vi "Test Open Close.vi"(8 "error in (no error)":errorcluster, 11 "Instrument.Oxford1820 in":refnum<class "Instrument.Oxford1820.lvclass">) -> (0 "error out":errorcluster, 3 "Instrument.Oxford1820 out":refnum<class "Instrument.Oxford1820.lvclass">)   [LabVIEW 2019, in "Instrument.Oxford1820.lvclass"]
uses:
  Instrument.Oxford1820.lvclass
  <instrlib>/Mercury iXX/Public/Libraries/Magnet/Controls/Device (Read).ctl
  <instrlib>/Mercury iXX/Public/Controls/Manufacturing Data.ctl
  <instrlib>/Mercury iXX/Public/Libraries/Magnet/Controls/Signals (Read).ctl
  Instrument.Oxford1820.lvclass/Instrument.Oxford1820.ctl
  <instrlib>/Mercury iXX/Public/Libraries/Magnet/Open/Open Magnet Device.vi
  <instrlib>/Mercury iXX/Public/Libraries/Magnet/Configuration/Read/Magnet Device (Read).vi
  <instrlib>/Mercury iXX/Mercury iXX.lvlib
  <instrlib>/Mercury iXX/Public/Libraries/Magnet.lvlib
panel:
  out "Magnet Device Details":T1={"Manufacturing"={"Hardware Version"="", "Firmware Version"="", "Serial Number"=""}, "Nickname"="", "Bipolar Output"="", "String"="SERS", "Current Limit"=0.0, "AtoB"=0.0, "Inductance"=0.0, "Switch Present"="", "Swh Htr Current"=0.0, "SW VLIM"=0.0, "V Trans Time"=0.0, "Magnet PSU Signals"={"Voltage"=0.0, "Current"=0.0, "Current Rate"=0.0, "Field"=0.0, "Field Rate"=0.0, "Persistant Current"=0.0, "Persistant Field"=0.0, "Target Current"=0.0, "Target Field"=0.0, "Target Current Rate"=0.0, "Target Field Rate"=0.0, "Switch Heater Status (SWHT)"="", "Switch Heater Status (SWHN)"=""}, "PSU Action"="SERS", "Status"="", "Level Limit"=0.0, "Temperature Limit"=0.0} {"Temperature Limit" format="%#.1f"; "Level Limit" format="%#.1f"; "V Trans Time" format="%#.1f"; "SW VLIM" format="%#.1f"; "Swh Htr Current" format="%#.1f"; "Inductance" format="%#.1f"; "AtoB" format="%#.1f"; "Current Limit" format="%#.1f"}
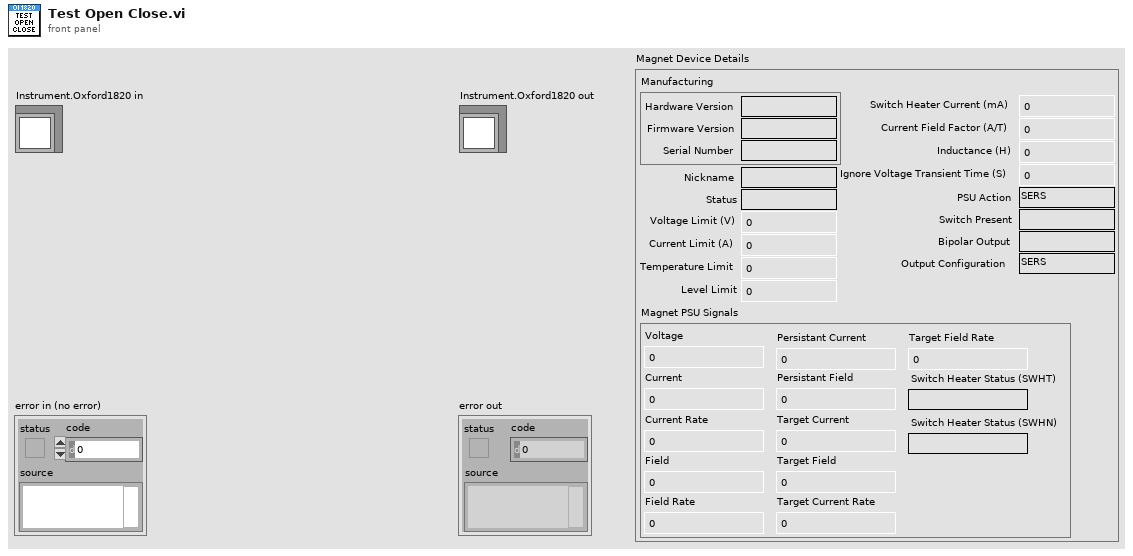
[diagram p1: front panel]
types:
  T1 = typedef "Mercury iXX.lvlib/Magnet.lvlib/Device (Read).ctl" = cluster{"Manufacturing":T2, "Nickname":string, "Bipolar Output":string, "String":string, "Current Limit":dbl, "AtoB":dbl, "Inductance":dbl, "Switch Present":string, "Swh Htr Current":dbl, "SW VLIM":dbl, "V Trans Time":dbl, "Magnet PSU Signals":T3, "PSU Action":string, "Status":string, "Level Limit":dbl, "Temperature Limit":dbl}
  T2 = typedef "Mercury iXX.lvlib/Manufacturing Data.ctl" = cluster{"Hardware Version":string, "Firmware Version":string, "Serial Number":string}
  T3 = typedef "Mercury iXX.lvlib/Magnet.lvlib/Signals (Read).ctl" = cluster{"Voltage":dbl, "Current":dbl, "Current Rate":dbl, "Field":dbl, "Field Rate":dbl, "Persistant Current":dbl, "Persistant Field":dbl, "Target Current":dbl, "Target Field":dbl, "Target Current Rate":dbl, "Target Field Rate":dbl, "Switch Heater Status (SWHT)":string, "Switch Heater Status (SWHN)":string}
  T4 = typedef "Mercury iXX.lvlib/Mercury Reference.ctl" = cluster{"Comms":refnum<visa-resource-name>, "Device ID":string[], "Comms Layer":T5, "Command":string, "Query reference":T6}
  T5 = typedef "Mercury iXX.lvlib/Comms Transport Layer.ctl" = enum16{"Ethernet TCP/IP", "USB", "ISOBus - RS-232", "GPIB"}
  T6 = typedef "Mercury iXX.lvlib/Query Dynamic Reference.ctl" = refnum<vi>
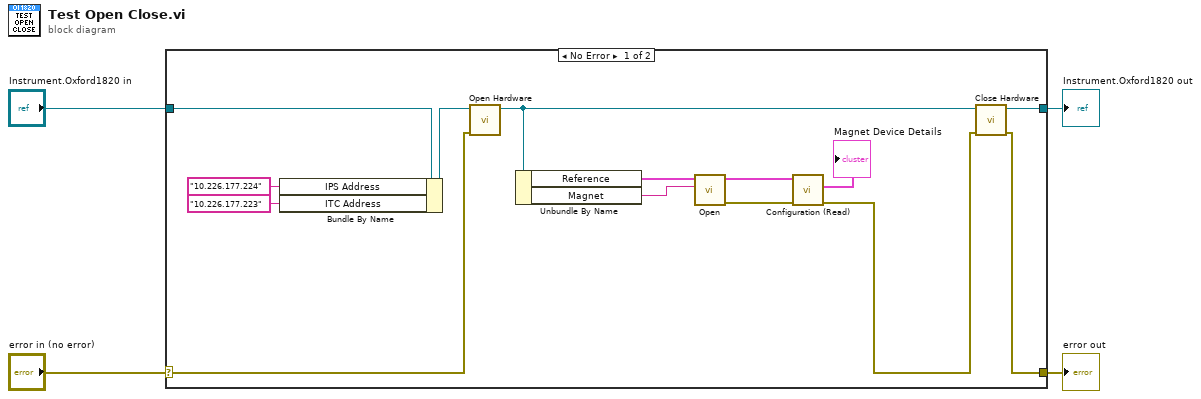
[diagram p0: block diagram]
diagram:
  n1 = case shown="No Error" "error in (no error)" {
    selector: "error in (no error)" -> [w17 w20]
    tunnel: [w16 w20] -> w3
    tunnel: [w18 w19] -> w1
    tunnel: "Instrument.Oxford1820 in" -> [w8 w19]
    frame No Error {
      n2 = Bundle By Name(cluster=w8, "IPS Address"="10.226.177.224" ("Configuration.IPS Address"), "ITC Address"="10.226.177.223" ("Configuration.ITC Address")) -> (w9:refnum<class "Instrument.Oxford1820.lvclass">)
      n3 = call-dynamic "Open Hardware.vi"("error in (no error)"=w17, "Instrument.Oxford1820 in"=w9) -> ("Instrument.Oxford1820 out"=w15:refnum<class "Instrument.Oxford1820.lvclass">)  [unwired: 8 in, 1 out]
      n4 = Unbundle By Name(w15) -> ("Reference"=w14:T4, "Magnet"=w10:string)
      n5 = call-poly <instrlib>:"Open.vi"("Device Identifier"=w10, "Mercury Reference In"=w14) -> ("error out"=w12:errorcluster, "Mercury Reference Out"=w13:T4)  [unwired: 8 in]
      n6 = call-poly <instrlib>:"Configuration (Read).vi"("error in"=w12, "Mercury Reference In"=w13) -> ("error out"=w5:errorcluster, "Magnet Device Details"=→"Magnet Device Details":T1)  [unwired: 6 in, 2 out]
      n7 = call-dynamic "Close Hardware.vi"("error in (no error)"=w5, "Instrument.Oxford1820 in"=w15) -> ("error out"=w16:errorcluster, "Instrument.Oxford1820 out"=w18:refnum<class "Instrument.Oxford1820.lvclass">)  [unwired: 8 in]
    }
    frame Error {
    }
  }
  "error out" <- w3
  "Instrument.Oxford1820 out" <- w1
